vi "Get Attribute.vi"(8 "error in (no error)":errorcluster, 10 "Name":string, 11 "AbstractData in":refnum<class "AbstractData.lvclass">) -> (0 "error out":errorcluster, 1 "value":variant, 2 "found":bool, 3 "AbstractData out":refnum<class "AbstractData.lvclass">)   [LabVIEW 2014, in "AbstractData.lvclass"]
uses:
  AbstractData.lvclass
  AbstractData.lvclass/AbstractData.ctl
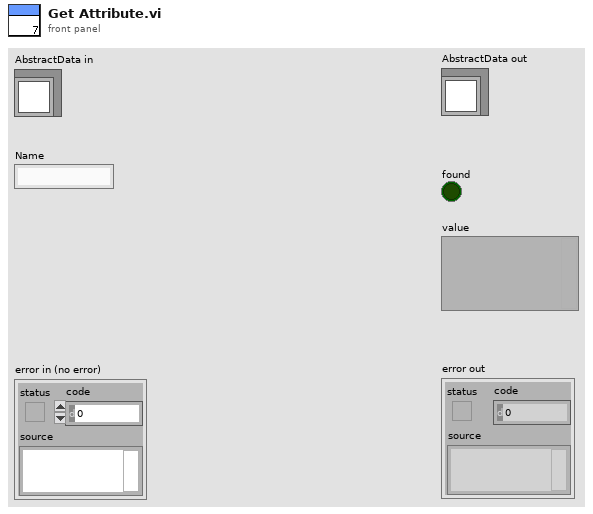
[diagram p1: front panel]
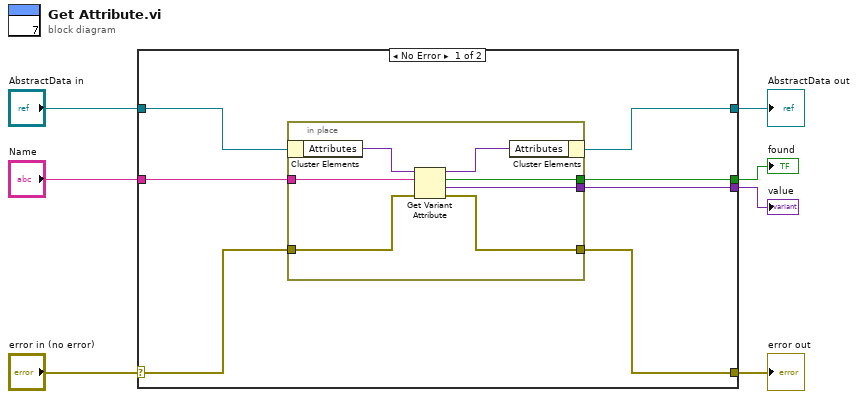
[diagram p0: block diagram]
diagram:
  n1 = case shown="No Error" "error in (no error)" {
    selector: "error in (no error)" -> [w12 w23]
    tunnel: [w11 w23] -> w6
    tunnel: [w13 w22] -> w4
    tunnel: "AbstractData in" -> [w14 w22]
    tunnel: [w10 _] -> w1
    tunnel: [w9 _] -> w2
    tunnel: "Name" -> [w8 _]
    frame No Error {
      n2 = in-place {
        in-place-border: w12 -> [w16]
        in-place-border: [w15] -> w11
        in-place-border: w8 -> [w19]
        in-place-border: [w18] -> w10
        in-place-border: [w17] -> w9
        n3 = in-place-cluster #1(w14) -> ("Attributes"=w21:variant)
        n4 = Get Variant Attribute(Variant=w21, name=w19, error in=w16) -> (duplicate Variant=w20:variant, found=w17:bool, value=w18:variant, error out=w15:errorcluster)  [unwired: 1 in]
        n5 = in-place-cluster #1("Attributes"=w20) -> (w13:refnum<class "AbstractData.lvclass">)
      }
    }
    frame Error {
    }
  }
  "error out" <- w6
  "AbstractData out" <- w4
  "found" <- w2
  "value" <- w1
